vi "append_to_image.vi"(8 "error in (no error)":errorcluster, 10 "data":dbl, 11 "scan_2d_hdf5_log in":refnum<class "scan_2d_hdf5_log.lvclass">) -> (0 "error out":errorcluster, 3 "scan_2d_hdf5_log out":refnum<class "scan_2d_hdf5_log.lvclass">)   [LabVIEW 2015, in "scan_2d_hdf5_log.lvclass"]
uses:
  scan_2d_hdf5_log.lvclass
  scan_2d_hdf5_log.lvclass/scan_2d_hdf5_log.ctl
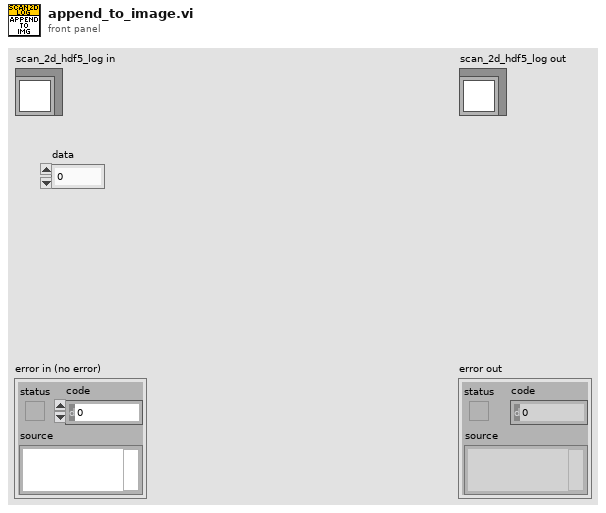
[diagram p1: front panel]
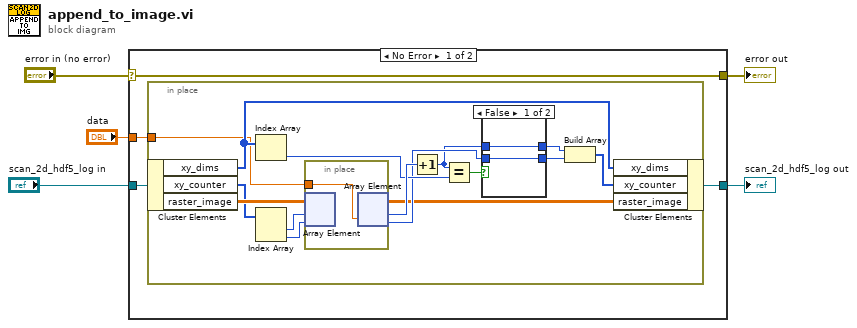
[diagram p0: block diagram]
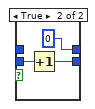
[diagram p2: hidden frame]
diagram:
  n1 = case shown="No Error" "error in (no error)" {
    selector: "error in (no error)" -> [w9 w32]
    tunnel: [w9 w32] -> w4
    tunnel: [w6 w31] -> w2
    tunnel: "scan_2d_hdf5_log in" -> [w8 w31]
    tunnel: "data" -> [w7 _]
    frame No Error {
      n2 = in-place {
        in-place-border: w7 -> [w12]
        n3 = in-place-cluster #1(w8) -> ("xy_dims"=w14:u32[], "xy_counter"=w23:i32[], "raster_image"=w24:dbl[][])
        n4 = Index Array(array=w14) -> (element=w19:u32)  [unwired: 1 in]
        n5 = Index Array(array=w23) -> (element #1=w22:i32, element #2=w10:i32)  [unwired: 2 in]
        n6 = in-place {
          in-place-border: w12 -> [w30]
          n7 = in-place-array #2(w24, w22, w10) -> ()  [unwired: 1 out]
          n8 = in-place-array #2(w30) -> (w11:dbl[][], w21:i32, w16:i32)
        }
        n9 = Increment(x=w21) -> (x+1=w13:i32)
        n10 = Equal?(x=w13, y=w19) -> (x = y?=w18:bool)
        n11 = case shown="False" w18 {
          tunnel: [w26 0 ("x+1")] -> w17
          tunnel: w16 -> [w25 w28]
          tunnel: [w25 w27] -> w15
          tunnel: w13 -> [w26 _]
          frame False {
          }
          frame True {
            n12 = Increment(x=w28) -> (x+1=w27:i32)
          }
        }
        n13 = Build Array(w17, w15) -> (w20:i32[])
        n14 = in-place-cluster #1("xy_dims"=w14, "xy_counter"=w20, "raster_image"=w11) -> (w6:refnum<class "scan_2d_hdf5_log.lvclass">)
      }
    }
    frame Error {
    }
  }
  "error out" <- w4
  "scan_2d_hdf5_log out" <- w2
